vi "Calculate Next Origin Point.vi"(8 "error in (no error)":errorcluster caption="错误输入（无错误）", 9 "origin":cluster{"x":i16, "y":i16} caption="Origin", 10 "Legend Info":T1={"Name"="", "Percent"=0.0, "TxtColor"=0, "Hor Space"=0, "Ver Space"=5, "Color Segement"=[16448250, 0, 16736786, 1198079]}, 11 "Gradient PieChart 输入":refnum<class "Gradient PieChart.lvclass"> caption="DNL_LabVIEW Object in") -> (0 "error out":errorcluster caption="错误输出", 2 "Next Origin":cluster{"x":i16, "y":i16} caption="Next Orgin", 3 "Gradient PieChart 输出":refnum<class "Gradient PieChart.lvclass"> caption="DNL_LabVIEW Object out")   [LabVIEW 2012, in "Gradient PieChart.lvclass"]
uses:
  Gradient PieChart.lvclass
  Legend Info.ctl
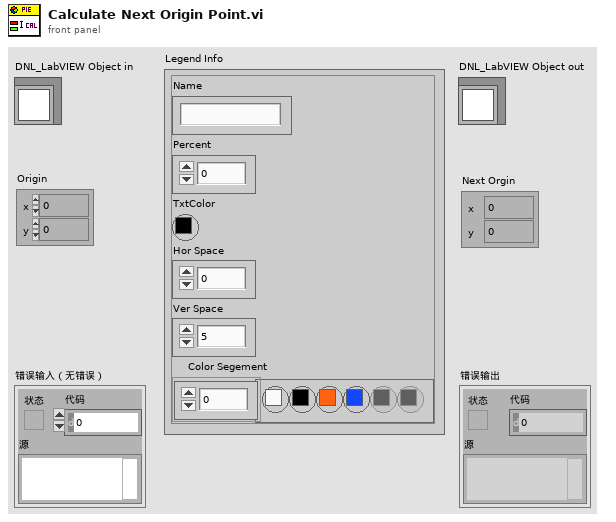
[diagram p1: front panel]
types:
  T1 = typedef "Gradient PieChart.lvclass/Legend Info.ctl" = cluster{"Name":string, "Percent":dbl, "TxtColor":u32, "Hor Space":i16, "Ver Space":i16, "Color Segement":u32[]}
  T2 = cluster{"left":i16, "top":i16, "right":i16, "bottom":i16}
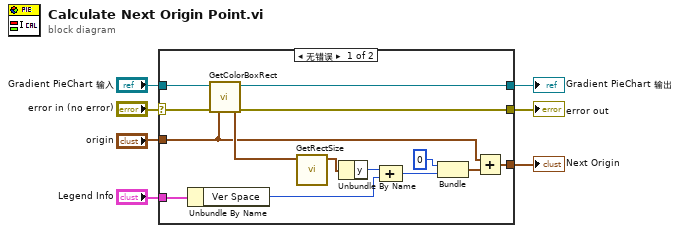
[diagram p0: block diagram]
diagram:
  n1 = case shown="无错误" "error in (no error)" {
    selector: "error in (no error)" -> [w18 w23]
    tunnel: [w17 w23] -> w6
    tunnel: [w19 w22] -> w4
    tunnel: "Gradient PieChart 输入" -> [w20 w22]
    tunnel: "Legend Info" -> [w21 _]
    tunnel: "origin" -> [w9 _]
    tunnel: [w8 _] -> w1
    frame No Error {
      n2 = Unbundle By Name(w21) -> ("Ver Space"=w13:i16)
      n3 = call "GetColorBoxRect.vi"("error in (no error)"=w18, "origin"=w9, "Gradient PieChart 输入"=w20) -> ("error out"=w17:errorcluster, "ColorBoxRect"=w16:T2, "Gradient PieChart 输出"=w19:refnum<class "Gradient PieChart.lvclass">)  [unwired: 6 in]
      n4 = call "GetRectSize.vi"("rect"=w16) -> ("point"=w15:cluster{"x":i16, "y":i16})  [unwired: 7 in, 3 out]
      n5 = Unbundle By Name(w15) -> ("y"=w14:i16)
      n6 = Compound Arithmetic op=ADD(w14, w13) -> (w12:i16)
      n7 = Bundle(i16 0, w12) -> (w10:cluster{i16, i16})  [unwired: 1 in]
      n8 = Add(x=w9, y=w10) -> (x+y=w8:cluster{i16, i16})
    }
    frame Error {
    }
  }
  "error out" <- w6
  "Gradient PieChart 输出" <- w4
  "Next Origin" <- w1
